vi "Autonomous Independent.vi"   [LabVIEW 2020]
doc: "This VI is called when autonomous begins, and will automatically be terminated when autonomous ends. You can carry out timed or sensor driven robot movement independently without needing to return to the caller."
uses:
  <vilib>/Rock Robotics/WPI/DriverStation/WPI_DriverStationAllianceInfo.ctl
  Arm/ArmPositionPreset.ctl
  Arm/ArmGamePiecePreset.ctl
  <vilib>/Rock Robotics/Network Tables/NT Read String.vi
  <vilib>/Rock Robotics/Network Tables/NT Write String.vi
  <vilib>/Rock Robotics/Network Tables/NT Read Integer.vi
  <vilib>/Rock Robotics/Network Tables/NT Read Number.vi
panel:
  # "Be sure to right-click and choose Data Operations>>Make Current Value default if you want to save the array values with the VI"
types:
  T1 = typedef "WPI_DriverStationAllianceInfo.ctl" = enum16{"Red", "Blue", "Invalid"}
  T2 = typedef "ArmGamePiecePreset.ctl" = enum16{"Cube", "Cone"}
  T3 = typedef "ArmPositionPreset.ctl" = enum16{"Upper", "Lower", "Middle", "Home", "Shelf", "Floor"}
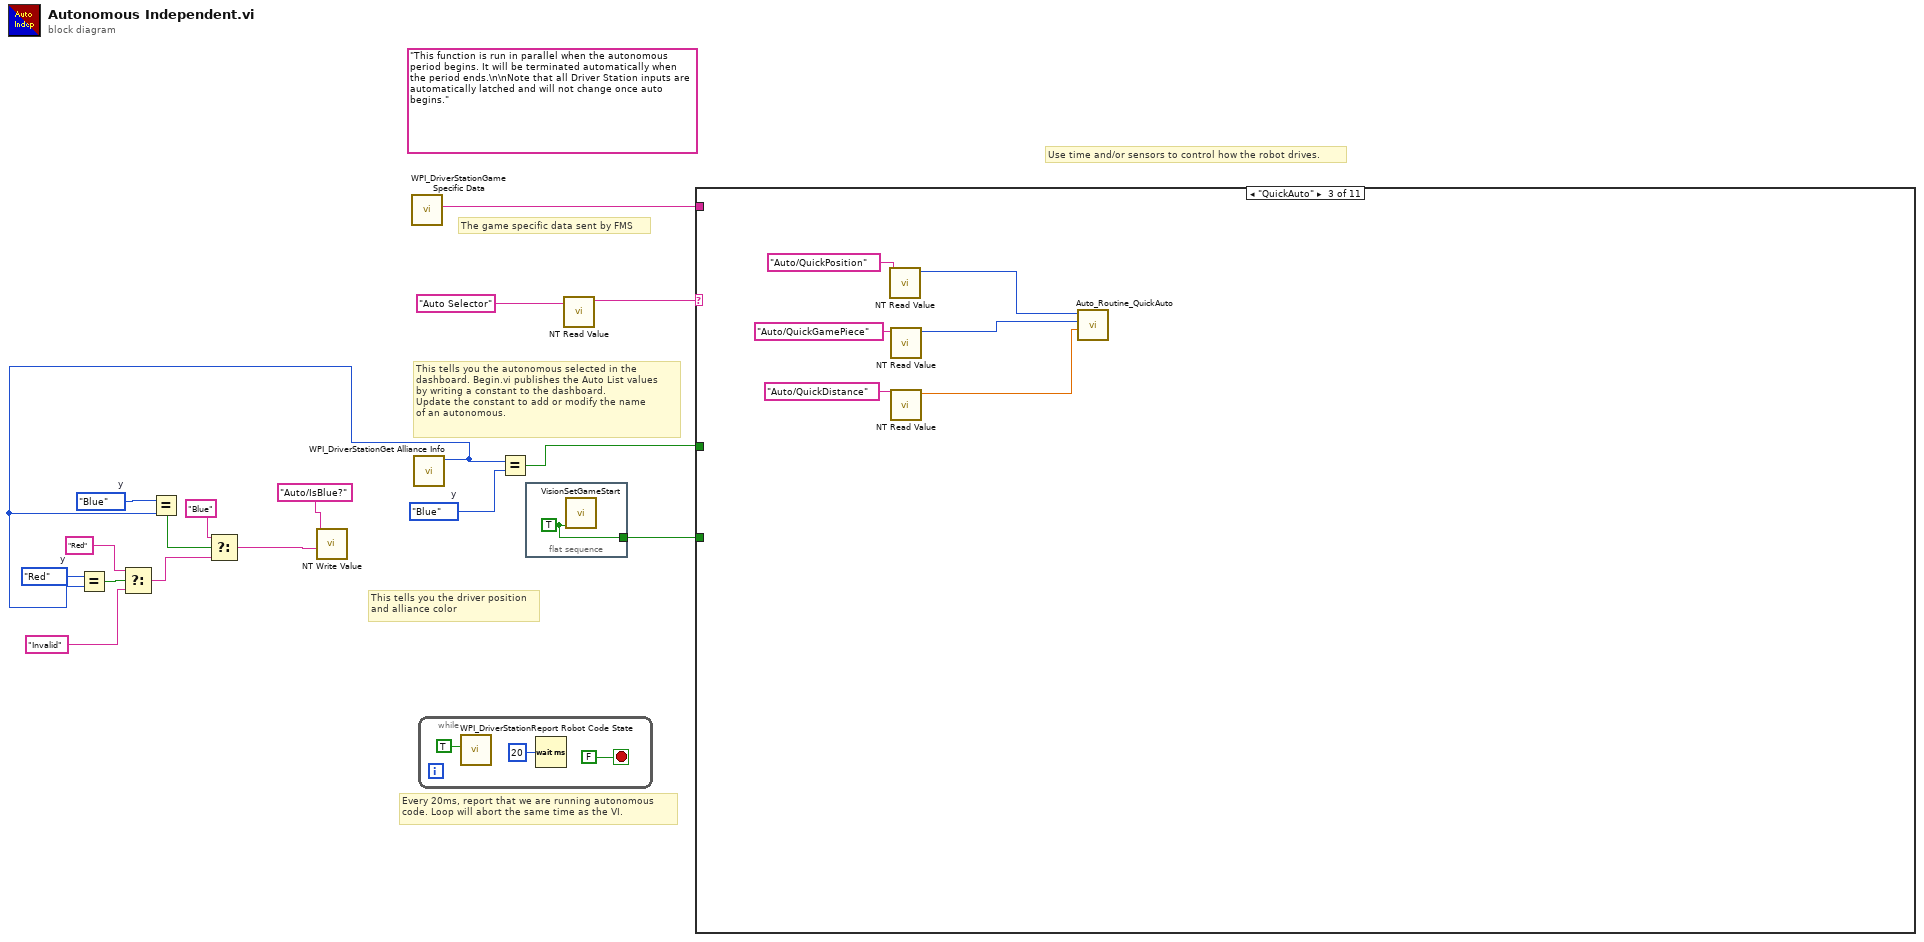
[diagram p0: block diagram]
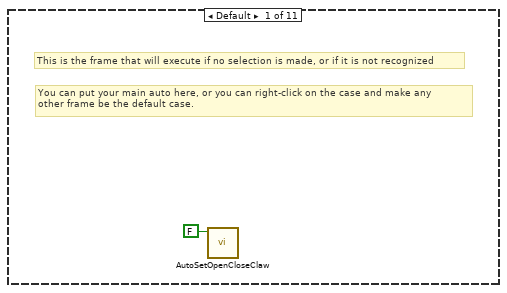
[diagram p2: hidden frame]
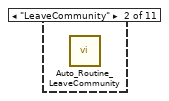
[diagram p3: hidden frame]
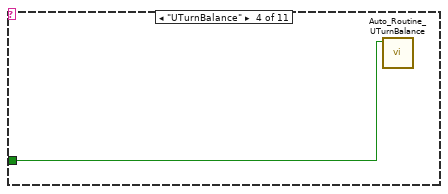
[diagram p4: hidden frame]
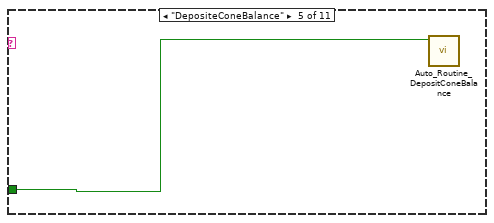
[diagram p5: hidden frame]
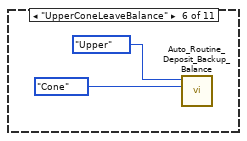
[diagram p6: hidden frame]
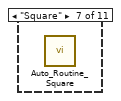
[diagram p7: hidden frame]
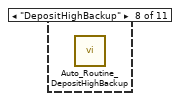
[diagram p8: hidden frame]
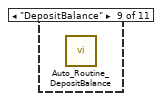
[diagram p9: hidden frame]
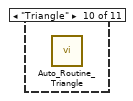
[diagram p10: hidden frame]
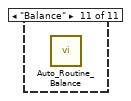
[diagram p11: hidden frame]
diagram:
  w9 = WPI_DriverStationAllianceInfo."Red"  # y
  w11 = WPI_DriverStationAllianceInfo."Blue"  # y
  w14 = WPI_DriverStationAllianceInfo."Blue"  # y
  (unwired) "This function is run in parallel when the autonomous period begins. It will be terminated automatically when the period ends.\n\nNote that all Driver Station inputs are automatically latched and will not change once auto begins."
  # "The game specific data sent by FMS"
  # "This tells you the autonomous selected in the \ndashboard. Begin.vi publishes the Auto List values\nby writing a constant to the dashboard.\nUpdate the constant to add or modify the name\nof an autonomous."
  # "Every 20ms, report that we are running autonomous\ncode. Loop will abort the same time as the VI."
  # "Use time and/or sensors to control how the robot drives."
  # "This tells you the driver position\nand alliance color"
  n1 = call <vilib>:"WPI_DriverStationGame Specific Data.vi"() -> ("Game Specific Data"=w15:string)  [unwired: 11 in]
  n2 = call <vilib>:"WPI_DriverStationGet Alliance Info.vi"() -> ("Alliance"=w3:T1)  [unwired: 11 out]
  n3 = Equal?(x=w9, y=w3) -> (x = y?=w8:bool)
  n4 = Select(t="Red", s=w8, f="Invalid") -> (s? t:f=w12:string)
  n5 = Equal?(x=w11, y=w3) -> (x = y?=w10:bool)
  n6 = Select(t="Blue", s=w10, f=w12) -> (s? t:f=w4:string)
  n7 = call-poly <vilib>:"NT Write Value.vi"("value"=w4, "name"="Auto/IsBlue?") -> ()  [unwired: 9 in, 1 out]
  n8 = while {
    stop <- FALSE stop-if-true
    n9 = call <vilib>:"WPI_DriverStationReport Robot Code State.vi"("Autonomous"=TRUE) -> ()  [unwired: 10 in, 1 out]
    n10 = Wait (ms)(milliseconds to wait=u32 20) -> ()  [unwired: 1 out]
  }
  n11 = Equal?(x=w3, y=w14) -> (x = y?=w2:bool)
  n12 = flat-sequence {
    tunnel: [w21] -> w1
    frame #0 {
      w21 = TRUE ("Game Start")
      n13 = call "VisionSetGameStart.vi"("Game Start"=w21) -> ()  [unwired: 11 in]
    }
  }
  n14 = call-poly <vilib>:"NT Read Value.vi"("name"="Auto Selector" ("Name")) -> ("value"=w16:string)  [unwired: 8 in, 2 out]
  n15 = case shown="\"QuickAuto\"" w16 {
    tunnel: w15 -> [_ _ _ _ _ _ _ _ _ _ _]
    tunnel: w2 -> [_ _ _ w29 w30 _ _ _ _ _ _]
    tunnel: w1 -> [_ _ _ _ _ _ _ _ _ _ _]
    frame Default {
      # "You can put your main auto here, or you can right-click on the case and make any\nother frame be the default case."
      # "This is the frame that will execute if no selection is made, or if it is not recognized"
      n16 = call "AutoSetOpenCloseClaw.vi"("Open?"=FALSE) -> ()  [unwired: 10 in, 1 out]
    }
    frame "LeaveCommunity" {
      n17 = call "Auto_Routine_LeaveCommunity.vi"() -> ()  [unwired: 11 in, 1 out]
    }
    frame "QuickAuto" {
      n18 = call-poly <vilib>:"NT Read Value.vi"("name"="Auto/QuickPosition") -> ("value"=w27:i64)  [unwired: 8 in, 2 out]
      n19 = call-poly <vilib>:"NT Read Value.vi"("name"="Auto/QuickGamePiece") -> ("value"=w26:i64)  [unwired: 8 in, 2 out]
      n20 = call-poly <vilib>:"NT Read Value.vi"("name"="Auto/QuickDistance") -> ("value"=w28:dbl)  [unwired: 8 in, 2 out]
      n21 = call "Auto_Routine_QuickAuto.vi"("Distance(Back)"=w28, "Game Piece"=w26, "Position"=w27) -> ()  [unwired: 8 in, 1 out]
    }
    frame "UTurnBalance" {
      n22 = call "Auto_Routine_UTurnBalance.vi"("IsBlue?"=w29) -> ()  [unwired: 10 in, 1 out]
    }
    frame "DepositeConeBalance" {
      n23 = call "Auto_Routine_DepositConeBalance.vi"("IsBlue?"=w30) -> ()  [unwired: 10 in, 1 out]
    }
    frame "UpperConeLeaveBalance" {
      n24 = call "Auto_Routine_Deposit_Backup_Balance.vi"("Game Piece"=ArmGamePiecePreset."Cone", "Position"=ArmPositionPreset."Upper") -> ()  [unwired: 9 in, 1 out]
    }
    frame "Square" {
      n25 = call "Auto_Routine_Square.vi"() -> ()  [unwired: 11 in, 1 out]
    }
    frame "DepositHighBackup" {
      n26 = call "Auto_Routine_DepositHighBackup.vi"() -> ()  [unwired: 11 in, 1 out]
    }
    frame "DepositBalance" {
      n27 = call "Auto_Routine_DepositBalance.vi"() -> ()  [unwired: 11 in, 1 out]
    }
    frame "Triangle" {
      n28 = call "Auto_Routine_Triangle.vi"() -> ()  [unwired: 11 in, 1 out]
    }
    frame "Balance" {
      n29 = call "Auto_Routine_Balance.vi"() -> ()  [unwired: 11 in, 1 out]
    }
  }
